vi "HIOKI PW3390 Conf CH B.vi"   [LabVIEW 2009]
doc: "Sets and reads the functions related to the Motor Analysis Option's Channel B. CH C input can select either Pulses or Analog DC."
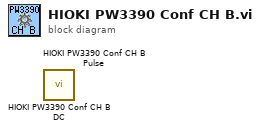
[diagram p0: block diagram]
diagram:
  n1 = call <instrlib>:"HIOKI PW3390 Conf CH B DC.vi"() -> ()  [unwired: 13 in, 7 out]
  n2 = call <instrlib>:"HIOKI PW3390 Conf CH B Pulse.vi"() -> ()  [unwired: 12 in, 8 out]
